vi "Reports.Translate Results V1 ZIP to JSON File With Data Files.vi"(7 "TempDir":path=path "C:/MTE/Translate/Temp", 10 "JSONOutDir":path, 11 "ZipFileIn":path) -> (0 "error out":errorcluster)   [LabVIEW 2018]
uses:
  <vilib>/KATE/Files/File Utils.lvlib
  <vilib>/zip/NI_Unzip.lvlib
  Results/Result.Measurement and Attribute Item Status.ctl
  Results/Result.Attribute.ctl
  Results/Result.Limit Type.ctl
  Results/Result.Numeric.ctl
  Results/Result XML/TestResult.Symptom.State.ctl
  Results/Result XML/TestResult.Symptom.ctl
  Results/Result XML/TestResult.UUT Result.ctl
  Results/Result XML/TestResult.Test Info.ctl
  Results/Result XML/TestResult.Test Run Info.ctl
  Results/Result XML/TestResult.SW Item.ctl
  Results/Result XML/TestResult.HW Item.ctl
  Results/Result XML/TestResult.Station Info.ctl
  Results/Result XML/TestResult.Facility.ctl
  Results/Result XML/TestResult.FullResultData.ctl
panel:
  out "Data Files":path[](array[path])
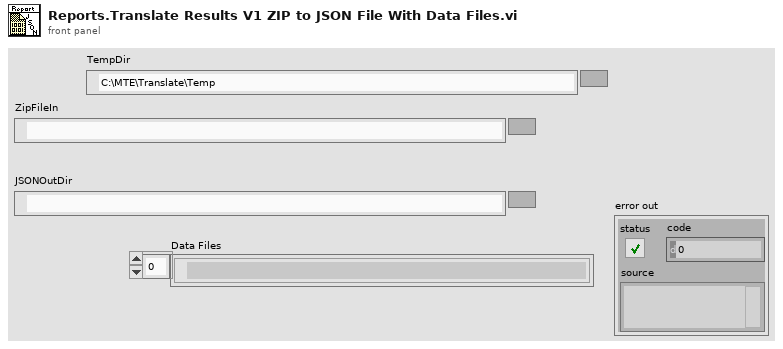
[diagram p1: front panel]
types:
  T1 = typedef "TestResult.FullResultData.ctl" = cluster{"#attributes":cluster{"Version":string}, "Facility":T2, "Station":T3, "Test Run":T6, "Test Sequence":T7, "UUTs":cluster{"UUT":T8[]}}
  T2 = typedef "TestResult.Facility.ctl" = cluster{"Name":string, "Location":string}
  T3 = typedef "TestResult.Station Info.ctl" = cluster{"Name":string, "PN":string, "SN":string, "Rev":string, "PC Name":string, "Location":string, "HW_Config":cluster{"HW_Item":T4[]}, "SW_Config":cluster{"SW_Item":T5[]}}
  T4 = typedef "TestResult.HW Item.ctl" = cluster{"Name":string, "MFG":string, "PN":string, "SN":string, "SW/FW":string, "Note":string, "Cal_ID":string, "Cal_Type":string, "Cal_Due_Date":timestamp, "Cal_Status":string}
  T5 = typedef "TestResult.SW Item.ctl" = cluster{"Name":string, "PN":string, "Version":string, "Note":string}
  T6 = typedef "TestResult.Test Run Info.ctl" = cluster{"Operator":string, "Start Time":timestamp, "Duration(s)":dbl, "Mode":string, "Comment":string, "ProcessStep":string}
  T7 = typedef "TestResult.Test Info.ctl" = cluster{"Name":string, "Config":cluster{"Config_Item":cluster{"Name":string, "Value":string}[]}}
  T8 = typedef "TestResult.UUT Info.ctl" = cluster{"Position":string, "PN":string, "SN":string, "Properties":cluster{"Property":cluster{"Name":string, "Value":string}[]}, "Result":T9, "Measurements":cluster{"Measurement":T11[]}, "Attributes":cluster{"Attribute":T14[]}}
  T9 = typedef "TestResult.Symptom.ctl" = cluster{"Result":T10, "Code":i32, "Description":string}
  T10 = typedef "TestResult.Symptom.State.ctl" = enum16{"Pass", "Fail", "Error", "Aborted", "Completed", "Logged"}
  T11 = typedef "Result.Numeric.ctl" = cluster{"Cnt":i32, "Step":string, "Category":string, "Name":string, "Value":dbl, "Units":string, "LimType":T12, "LL":dbl, "UL":dbl, "Status":T13, "Code":i32, "Desc":string, "Time":timestamp}
  T12 = typedef "Result.Limit Type.ctl" = enum16{"None", "EQ", "NE", "GT", "LT", "GE", "LE", "GTLT", "GELE", "GELT", "GTLE", "LTGT", "LEGE", "LEGT", "LTGE"}
  T13 = typedef "Result.Measurement and Attribute Item Status.ctl" = i32
  T14 = typedef "Result.Attribute.ctl" = cluster{"Cnt":i32, "Step":string, "Category":string, "Name":string, "Value":string, "Status":T13, "Code":i32, "Desc":string, "Time":timestamp}
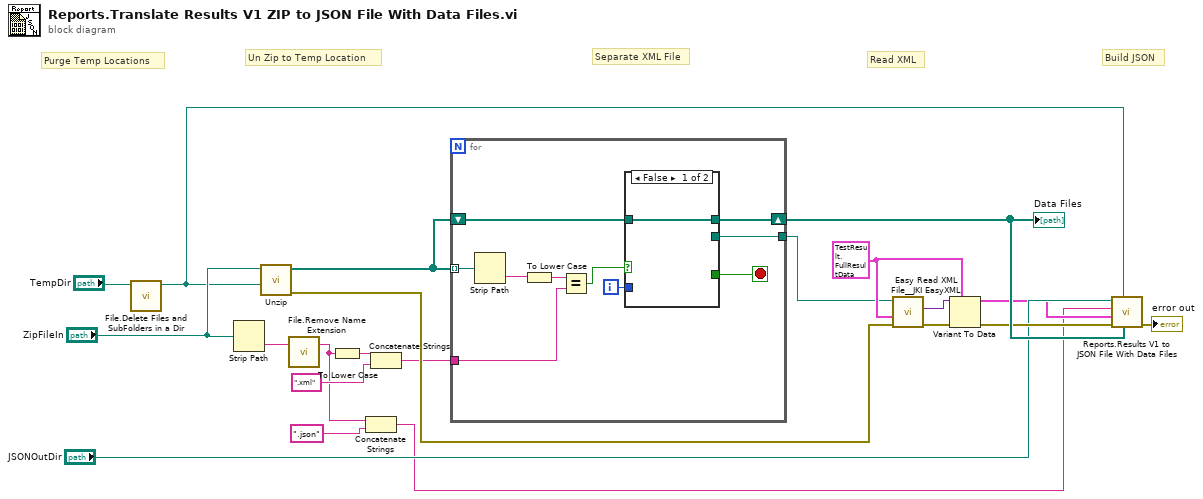
[diagram p0: block diagram]
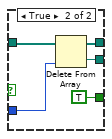
[diagram p2: hidden frame]
diagram:
  w16 = T1 {"#attributes"={"Version"="MTE_1.0.0"}, "Facility"={"Name"="", "Location"=""}, "Station"={"Name"="", "PN"="", "SN"="", "Rev"="", "PC Name"="", "Location"="", "HW_Config"={"HW_Item"=[]}, "SW_Config"={"SW_Item"=[]}}, "Test Run"={"Operator"="", "Start Time"=timestamp(0 s since 1904-01-01), "Duration(s)"=0.0, "Mode"="", "Comment"="", "ProcessStep"=""}, "Test Sequence"={"Name"="", "Config"={"Config_Item"=[]}}, "UUTs"={"UUT"=[]}} ("Test Result")
  # "Read XML"
  # "Purge Temp Locations"
  # "Build JSON"
  # "Un Zip to Temp Location"
  # "Separate XML File"
  n1 = call <vilib>:"File.Delete Files and SubFolders in a Dir.vi"("Dir"="TempDir") -> ("Dup Dir"=w6:path)  [unwired: 9 in, 1 out]
  n2 = Strip Path(path="ZipFileIn") -> (name=w8:string)  [unwired: 1 out]
  n3 = call <vilib>:"Unzip.vi"("Target directory (same as Zip file if empty)"=w6, "Zip file"="ZipFileIn") -> ("error out"=w15:errorcluster, "Unzipped files"=w14:path[])  [unwired: 7 in, 1 out]
  n4 = call <vilib>:"File.Remove Name Extension.vi"("File Name"=w8) -> ("Name Less Ext"=w3:string)  [unwired: 1 in, 1 out]
  n5 = To Lower Case(string=w3) -> (all lower case string=w20:string)
  n6 = Concatenate Strings(w3, ".json" ("string")) -> (w1:string)
  n7 = Concatenate Strings(w20, ".xml" ("string")) -> (w4:string)
  n8 = for {
    tunnel: w14 -> [w31] mode=indexing
    shift-right: [w29] -> w11
    shift-left: w14 -> [w30]
    tunnel: [w27] -> w13
    tunnel: w4 -> [w24]
    i -> [w28]
    stop <- w26 stop-if-true
    n9 = Strip Path(path=w31) -> (name=w22:string)  [unwired: 1 out]
    n10 = To Lower Case(string=w22) -> (all lower case string=w25:string)
    n11 = Equal?(x=w25, y=w24) -> (x = y?=w23:bool)
    n12 = case shown="False" w23 {
      tunnel: [_ TRUE] -> w26
      tunnel: w30 -> [w32 w36]
      tunnel: [w32 w35] -> w29
      tunnel: w28 -> [_ w33]
      tunnel: [_ w34] -> w27
      frame False {
      }
      frame True {
        n13 = Delete From Array(array=w36, index=w33) -> (deleted portion=w34:path, array with subset deleted=w35:path[])  [unwired: 1 in]
      }
    }
  }
  "Data Files" <- w11
  n14 = call <vilib>:"Easy Read XML File__JKI EasyXML.vi"("error in (no error)"=w15, "LabVIEW Data (Type)"=w16, "XML File Path"=w13) -> ("error out"=w18:errorcluster, "LabVIEW Data"=w17:variant)  [unwired: 6 in, 1 out]
  n15 = Variant To Data(error in=w18, type=w16, Variant=w17) -> (data=w7:T1, error out=w10:errorcluster)
  n16 = call "Reports.Results V1 to JSON File With Data Files.vi"("File Data Objs"=w11, "Temp Folder"=w6, "error in (no error)"=w10, "Test Result In"=w7, "File Name"=w1, "Folder"="JSONOutDir") -> ("error out"=→"error out":errorcluster)  [unwired: 5 in]
